vi "RetrieveProviderCotentVIPath.vi"(8 "error in (no error)":errorcluster) -> (0 "error out":errorcluster, 2 "Initialize-API":path)   [LabVIEW 2019, in "LabVIEW-ProviderShell.lvlib" / "LvProviderShellHelper.lvclass"]
uses:
  LvProviderShellHelper.lvclass
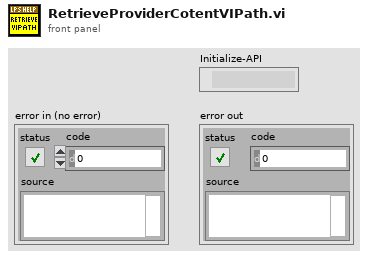
[diagram p1: front panel]
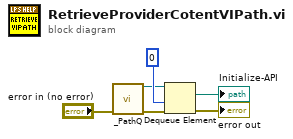
[diagram p0: block diagram]
diagram:
  n1 = call "_PathQ.vi"("error in (no error)"="error in (no error)") -> ("error out"=w1:errorcluster, "Queue out"=w2:refnum<queue>)  [unwired: 9 in]
  n2 = Dequeue Element(queue=w2, timeout in ms (-1)=0, error in (no error)=w1) -> (element=→"Initialize-API":path, error out=→"error out":errorcluster)  [unwired: 2 out]
